vi "Hit Test.vi"(10 "point":T1, 11 "Blob in":refnum<class "Blob.lvclass">) -> (2 "hit":bool)   [LabVIEW 2023, in "Blob.lvclass"]
doc: "See if the point is within the bounds of the blob."
uses:
  Blob.lvclass
  <vilib>/Utility/miscctls.llb/LVPoint32TypeDef.ctl
  Blob.lvclass/Blob.ctl
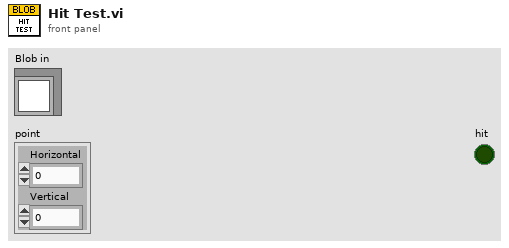
[diagram p1: front panel]
types:
  T1 = typedef "LVPoint32TypeDef.ctl" = cluster{"Horizontal":i32, "Vertical":i32}
  T2 = typedef "LVRectTypeDef.ctl" = cluster{"Left":i16, "Top":i16, "Right":i16, "Bottom":i16}
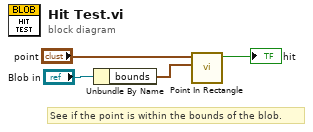
[diagram p0: block diagram]
diagram:
  # "See if the point is within the bounds of the blob."
  n1 = Unbundle By Name("Blob in") -> ("bounds"=w3:T2)
  n2 = call "Point In Rectangle.vi"("rect"=w3, "point"="point") -> ("point in rect"=→"hit":bool)  [unwired: 9 in]
